vi "SCD - Log Recipe Step Information.vi"(8 "error in (no error)":errorcluster, 9 "Arg 3":path, 10 "Data Type":T1, 11 "Recipe Step":i32=1) -> (0 "error out":errorcluster, 3 "Recipe Being Processed":string)   [LabVIEW 2014]
doc: "Use this template to build a VI to use as a subVI."
uses:
  Controls/Cbk Data type.ctl
panel:
  out "text":string
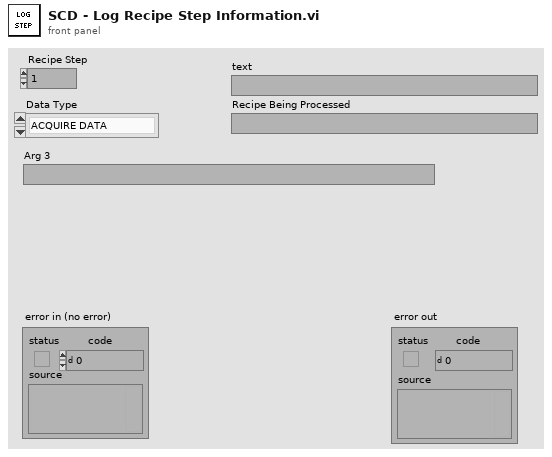
[diagram p1: front panel]
types:
  T1 = typedef "Cbk Data type.ctl" = enum32{"ACQUIRE DATA", "SET DIFFUSER", "CAL-FW", "WAVELENGTH-FW", "INSTR. ROTATION", "SET FOCUS", "DATATYPE", "SET EXPOSURE", "CBK COMMENTS", "MOVE-PI", "MOVE-PI2", "MOVE-PI3", "DWELL TIME"}
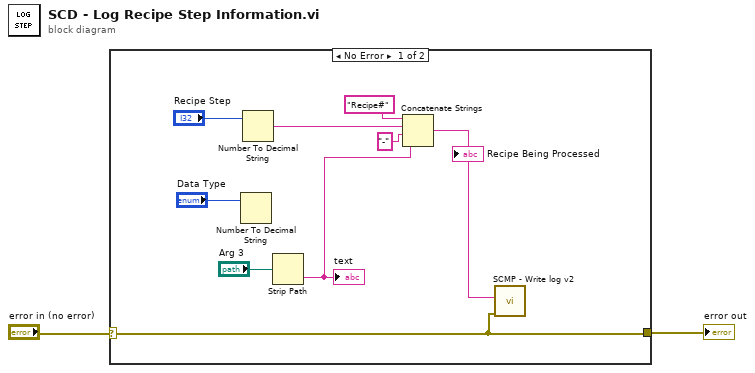
[diagram p0: block diagram]
diagram:
  n1 = case shown="No Error" "error in (no error)" {
    selector: "error in (no error)" -> [w3 w12]
    tunnel: [w3 w12] -> w2
    frame No Error {
      n2 = Number To Decimal String(number="Data Type") -> ()  [unwired: 1 in, 1 out]
      n3 = Number To Decimal String(number="Recipe Step") -> (decimal integer string=w7:string)  [unwired: 1 in]
      n4 = Strip Path(path="Arg 3") -> (name=w5:string)  [unwired: 1 out]
      "text" <- w5
      n5 = Concatenate Strings("Recipe#" ("string"), w7, "-" ("string"), w5) -> (w10:string)
      "Recipe Being Processed" <- w10
      n6 = call "SCMP - Write log v2.vi"("Error to log"=w3, "data"=w10) -> ()  [unwired: 7 in, 3 out]
    }
    frame Error {
    }
  }
  "error out" <- w2
